vi "New SenseHat.Joystick.vi"(8 "error in (no error)":errorcluster, 11 "SenseHat in":refnum<class "SenseHat.lvclass">) -> (0 "error out":errorcluster, 3 "SenseHat out":refnum<class "SenseHat.lvclass">)   [LabVIEW 2020, in "RPI.SenseHat.lvlib" / "SenseHat.lvclass"]
uses:
  SenseHat.lvclass
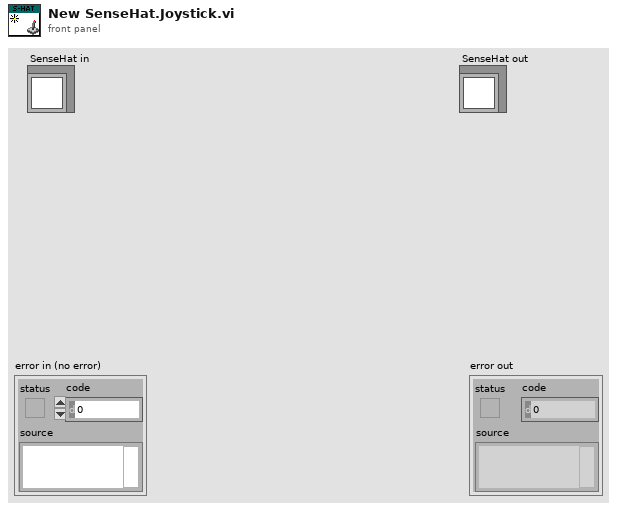
[diagram p1: front panel]
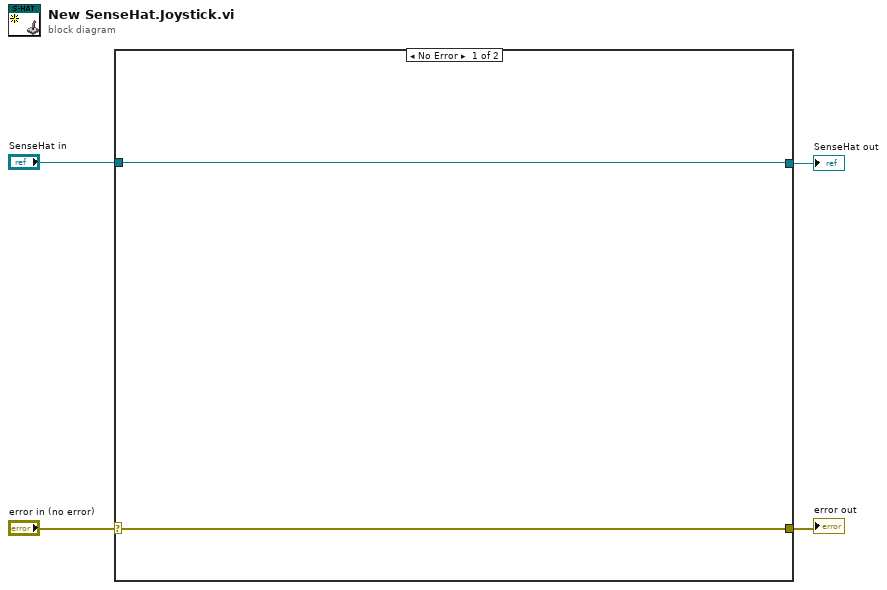
[diagram p0: block diagram]
diagram:
  n1 = case shown="No Error" "error in (no error)" {
    selector: "error in (no error)" -> [w6 w8]
    tunnel: [w6 w8] -> w3
    tunnel: [w5 w7] -> w1
    tunnel: "SenseHat in" -> [w5 w7]
    frame No Error {
    }
    frame Error {
    }
  }
  "error out" <- w3
  "SenseHat out" <- w1
